vi "Example - Logger.vi"() -> ()   [LabVIEW 2021, in "F-70 driver.lvlib"]
uses:
  F-70 driver.lvlib
panel:
  in  "logging interval (s)":dbl=5000.0
  out "State of operation":u16(ring) items=["Local Off", "Local On", "Remote Off", "Remote On", "Cold head Run", "Cold head pause", "Fault Off", "Oil Fault Off"]
  in  "Stop":bool
  in  "VISA resource in":refnum<visa-resource-name>="COM4"
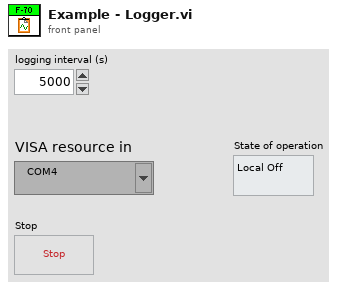
[diagram p1: front panel]
types:
  T1 = enum16{"open", "replace", "create", "open or create", "replace or create", "replace or create with confirmation"}
  T2 = typedef "F-70 driver.lvlib/F-70 parameters.ctl" = cluster{"FW version":dbl, "Elapsed hours":dbl, "He discharge Tmp (°C)":dbl, "Water out Tmp (°C)":dbl, "Water in Tmp (°C)":dbl, "Return pressure (PSIG)":dbl, "Configuration":bool, "State of operation":u16, "Solenoid":bool, "Pressure alarm":bool, "Oil level alarm":bool, "Water flow alarm":bool, "Water Tmp alarm":bool, "He Tmp alarm":bool, "Fuse alarm":bool, "Motor Tmp alarm":bool, "System":bool, "Last updated":timestamp, "Last response":string}
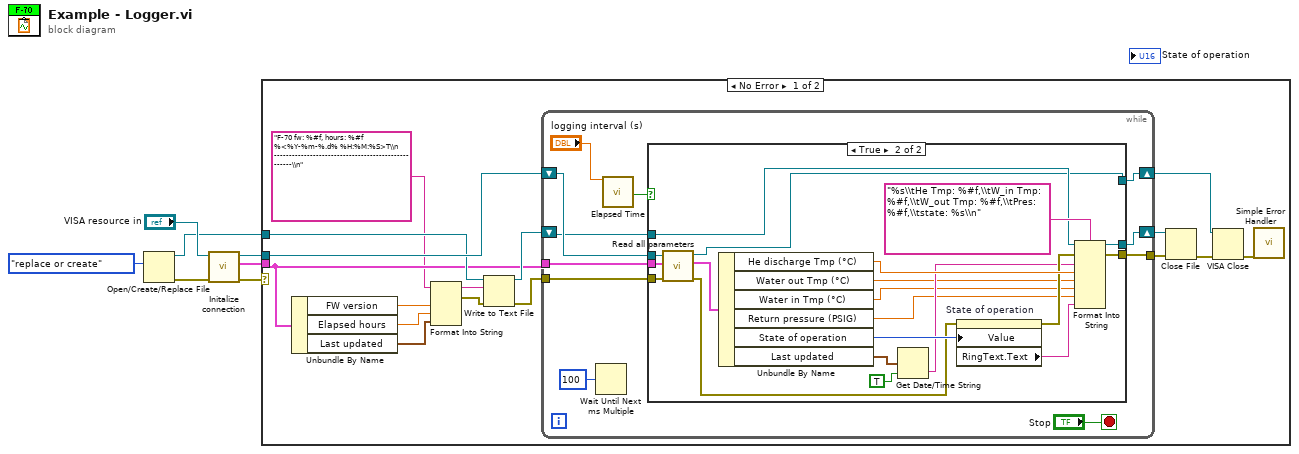
[diagram p0: block diagram]
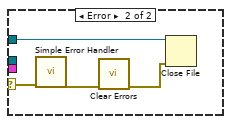
[diagram p3: hidden frame]
diagram:
  n1 = Open/Create/Replace File(operation (0:open)=T1."replace or create") -> (refnum out=w1:refnum<file>, error out=w3:errorcluster)  [unwired: 5 in, 1 out]
  n2 = call "Initalize connection.vi"("error in (no error)"=w3, "VISA resource in"="VISA resource in") -> ("error out"=w2:errorcluster, "F-70 parameters out"=w5:T2, "VISA resource out"=w6:refnum<visa-resource-name>)  [unwired: 3 in]
  n3 = case shown="No Error" w2 {
    selector: w2 -> [_ w61]
    tunnel: w6 -> [w23 _]
    tunnel: w5 -> [w19 _]
    tunnel: w1 -> [w22 w60]
    frame No Error {
      n4 = Unbundle By Name(w19) -> ("FW version"=w18:dbl, "Elapsed hours"=w17:dbl, "Last updated"=w13:timestamp)
      n5 = Format Into String(format string="F-70 fw: %#f, hours: %#f %<%Y-%m-%.d% %H:%M:%S>T\\n ---------------------------------------------------\\n", w18, w17, w13) -> (resulting string=w15:string, error out=w14:errorcluster)  [unwired: 2 in]
      n6 = Write to Text File(file (use dialog)=w22, text=w15, error in=w14) -> (refnum out=w21:refnum<file>, error out=w20:errorcluster)  [unwired: 1 in, 1 out]
      n7 = while {
        tunnel: w19 -> [w33]
        tunnel: w20 -> [w31]
        tunnel: [w28] -> w11
        shift-right: [w29] -> w12
        shift-left: w21 -> [w30]
        shift-right: [w27] -> w8
        shift-left: w23 -> [w32]
        stop <- "Stop" stop-if-true
        n8 = Wait Until Next ms Multiple(millisecond multiple=u32 100) -> ()  [unwired: 1 out]
        n9 = call "Elapsed Time"("Time Target (s)"="logging interval (s)") -> ("Time has Elapsed"=w25:bool)  [unwired: 11 in, 7 out]
        n10 = case shown="True" w25 {
          tunnel: w33 -> [_ w57]
          tunnel: w32 -> [w37 w56]
          tunnel: w31 -> [w35 w54]
          tunnel: w30 -> [w36 w45]
          tunnel: [w36 w44] -> w29
          tunnel: [w35 w43] -> w28
          tunnel: [w37 w38] -> w27
          frame False {
          }
          frame True {
            n11 = call "Read all parameters.vi"("error in"=w54, "F-70 parameters in"=w57, "VISA resource in"=w56) -> ("error out"=w47:errorcluster, "F-70 parameters in 2"=w55:T2, "VISA resource out"=w38:refnum<visa-resource-name>)  [unwired: 2 in]
            n12 = Unbundle By Name(w55) -> ("He discharge Tmp (°C)"=w50:dbl, "Water out Tmp (°C)"=w39:dbl, "Water in Tmp (°C)"=w40:dbl, "Return pressure (PSIG)"=w41:dbl, "State of operation"=w49:u16, "Last updated"=w52:timestamp)
            n13 = Get Date/Time String(seconds (now)=w52, want seconds? (F)=TRUE) -> (time string=w46:string)  [unwired: 1 in, 1 out]
            n14 = property on="State of operation" class="Ring (strict)"(error in=w47, "Value"=w49) -> (error out=w48:errorcluster, "RingText.Text"=w42:string)  [unwired: 1 in, 1 out]
            n15 = Format Into String(format string="%s\\tHe Tmp: %#f,\\tW_in Tmp: %#f,\\tW_out Tmp: %#f,\\tPres: %#f,\\tstate: %s\\n", initial string=w45, error in=w48, w46, w50, w39, w40, w41, w42) -> (resulting string=w44:refnum<file>, error out=w43:errorcluster)
          }
        }
      }
      n16 = Close File(refnum=w12, error in=w11) -> (error out=w10:errorcluster)  [unwired: 1 out]
      n17 = VISA Close(VISA resource name=w8, error in (no error)=w10) -> (error out=w9:errorcluster)
      n18 = call <vilib>:"Simple Error Handler.vi"("error in (no error)"=w9) -> ()  [unwired: 4 in, 5 out]
    }
    frame Error {
      n19 = call <vilib>:"Simple Error Handler.vi"("error in (no error)"=w61) -> ("error out"=w58:errorcluster)  [unwired: 4 in, 4 out]
      n20 = call <vilib>:"Clear Errors.vi"("error in (no error)"=w58) -> ("error out"=w59:errorcluster)  [unwired: 5 in, 1 out]
      n21 = Close File(refnum=w60, error in=w59) -> ()  [unwired: 2 out]
    }
  }
